vi "UpdateMCS.vi"(0 "Show MCS":bool, 1 "Retrace":bool, 2 "Update Data":T1, 3 "MCS Trace":refnum<vi>) -> ()   [LabVIEW 2009]
panel:
  in  "Boolean":bool
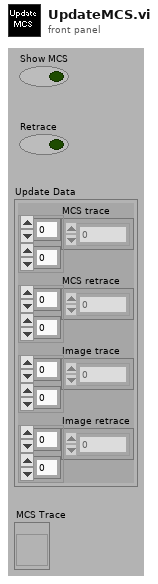
[diagram p1: front panel]
types:
  T1 = cluster{"MCS trace":u32[][], "MCS retrace":u32[][], "Image trace":u32[][], "Image retrace":u32[][]}
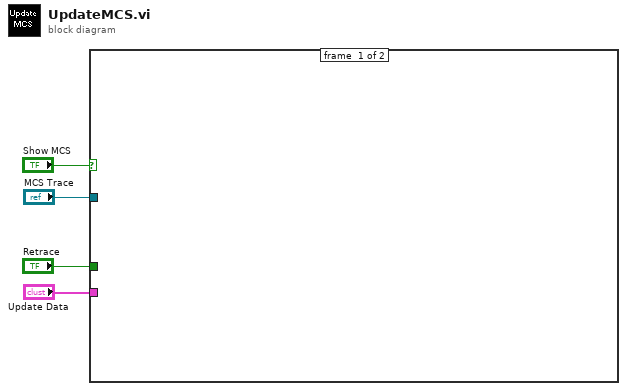
[diagram p0: block diagram]
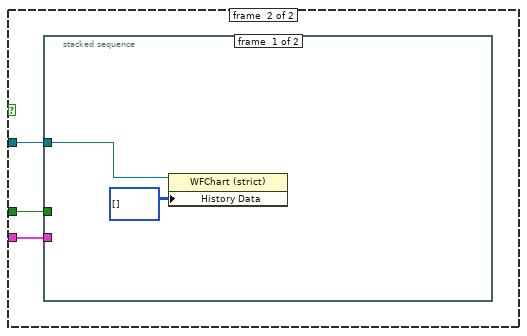
[diagram p2: hidden frame]
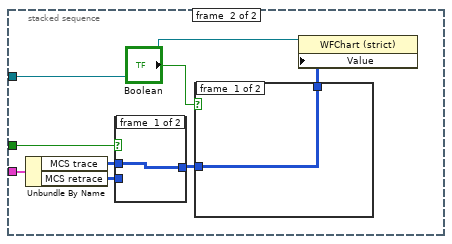
[diagram p3: hidden frame]
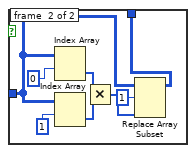
[diagram p4: hidden frame]
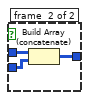
[diagram p5: hidden frame]
diagram:
  n1 = case shown="True" "Show MCS" {
    tunnel: "MCS Trace" -> [_ w5]
    tunnel: "Update Data" -> [_ w7]
    tunnel: "Retrace" -> [_ w6]
    frame #0 {
    }
    frame #1 {
      n2 = stacked-sequence {
        tunnel: w7 -> [_ w17]
        tunnel: w6 -> [_ w16]
        tunnel: w5 -> [w8 w15]
        frame #0 {
          n3 = property class="WFChart (strict)"(reference=w8, "History Data"=u32[][] []) -> ()  [unwired: 1 in, 2 out]
        }
        frame #1 {
          n4 = Unbundle By Name(w17) -> ("MCS trace"=w14:u32[][], "MCS retrace"=w13:u32[][])
          n5 = case shown="False" w16 {
            tunnel: w14 -> [w27 w30]
            tunnel: w13 -> [_ w29]
            tunnel: [w27 w28] -> w12
            frame #0 {
            }
            frame #1 {
              n6 = Build Array (concatenate)(w30, w29) -> (w28:u32[][])
            }
          }
          n7 = case shown="True" "Boolean" {
            tunnel: w12 -> [w18 w22]
            tunnel: [w18 w19] -> w11
            frame #0 {
            }
            frame #1 {
              n8 = Index Array(array=w22, index (row)=0 ("index")) -> (element=w24:u32[])  [unwired: 1 in]
              n9 = Index Array(array=w22, index (row)=1 ("index")) -> (element=w23:u32[])  [unwired: 1 in]
              n10 = Multiply(x=w24, y=w23) -> (x*y=w21:u32[])
              n11 = Replace Array Subset(array=w22, new element=w21, index (row)=1) -> (w19:u32[][])  [unwired: 1 in]
            }
          }
          n12 = property class="WFChart (strict)"(reference=w15, "Value"=w11) -> ()  [unwired: 1 in, 2 out]
        }
      }
    }
  }
